vi "Control_3.vi"(0 "latd-lon-heig-VNWU":T5, 1 "CIVITA as DMARS [rad]":cluster{"phi":dbl, "theta":dbl, "psi":dbl}, 2 "Guiamento":bool, 3 "PID_array":dbl[][](array[numeric]), 5 "Wi1-Wbi1-qi1-Euli1":T6, 7 "Civita?":bool, 9 "output Rocket Dynamics":T1, 11 "File":dbl[][](array[numeric]), 12 "dt-sim_run-t-i":T4, 13 "Position (i+1)":T2, 14 "Rotation":T3, 15 "sim_running":bool) -> (4 "TVA_cmd(i+1,:) [deg]":dbl[](array[numeric]), 10 "AoA-Speed-Rocket":cluster{dbl[], dbl[], dbl[]})   [LabVIEW 2017]
uses:
  <vilib>/Analysis/coordinate.llb/Euler Rotation Order.ctl
  <vilib>/Analysis/_algsub.llb/Vector Norm Type.ctl
  <vilib>/Analysis/baseanly.llb/Real A x B.vi
  <vilib>/Analysis/_algsub.llb/Real Vector Norm.vi
  <vilib>/Analysis/Matrix/Numeric/Conversions/Array To Matrix - RA2.vi
  <vilib>/Analysis/Matrix/Numeric/Conversions/Matrix To Array - RM.vi
  <vilib>/Analysis/NI_AALPro.lvlib
  <vilib>/Analysis/Matrix/NI_Matrix.lvlib
  <vilib>/Analysis/NI_AALBase.lvlib
panel:
  out "Pitch Yaw ref [deg]":dbl[](array[numeric])
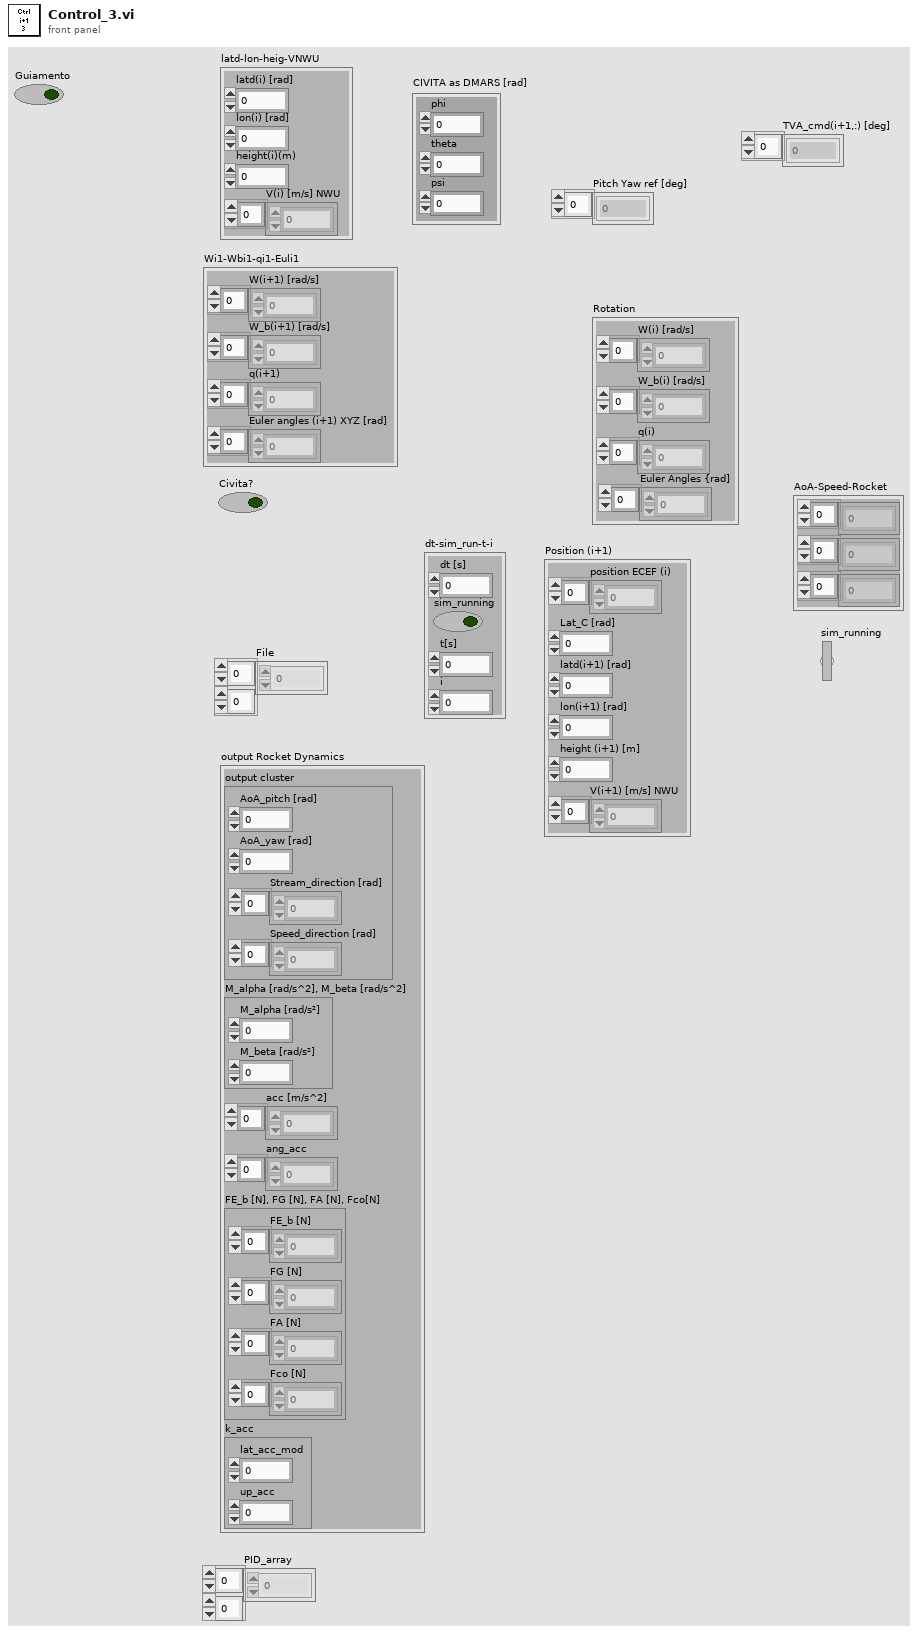
[diagram p1: front panel]
types:
  T1 = cluster{"output cluster":cluster{"AoA_pitch [rad]":dbl, "AoA_yaw [rad]":dbl, "Stream_direction [rad]":dbl[], "Speed_direction [rad]":dbl[]}, "M_alpha [rad/s^2], M_beta [rad/s^2]":cluster{"M_alpha [rad/s²]":dbl, "M_beta [rad/s²]":dbl}, "acc [m/s^2]":dbl[], "ang_acc":dbl[], "FE_b [N], FG [N], FA [N], Fco[N]":cluster{"FE_b [N]":dbl[], "FG [N]":dbl[], "FA [N]":dbl[], "Fco [N]":dbl[]}, "k_acc":cluster{"lat_acc_mod":dbl, "up_acc":dbl}}
  T2 = cluster{"position ECEF (i)":dbl[], "Lat_C [rad]":dbl, "latd(i+1) [rad]":dbl, "lon(i+1) [rad]":dbl, "height (i+1) [m]":dbl, "V(i+1) [m/s] NWU":dbl[]}
  T3 = cluster{"W(i) [rad/s]":dbl[], "W_b(i) [rad/s]":dbl[], "q(i)":dbl[], "Euler Angles {rad]":dbl[]}
  T4 = cluster{"dt [s]":dbl, "sim_running":bool, "t[s]":dbl, "i":i32}
  T5 = cluster{"latd(i) [rad]":dbl, "lon(i) [rad]":dbl, "height(i)(m)":dbl, "V(i) [m/s] NWU":dbl[]}
  T6 = cluster{"W(i+1) [rad/s]":dbl[], "W_b(i+1) [rad/s]":dbl[], "q(i+1)":dbl[], "Euler angles (i+1) XYZ [rad]":dbl[]}
  T7 = enum16{"IPD_deg_labview", "PID_deg_labview", "old 2019", "PID tunner", "VS 50 Control System database doc"}
  T8 = typedef "NI_AALPro.lvlib/Vector Norm Type.ctl" = u16
  T9 = typedef "NI_AALPro.lvlib/Euler Rotation Order.ctl" = u16
  T10 = typedef "NI_Matrix.lvlib/RealMatrix.ctl" = dbl[][]
  T11 = cluster{"M_alpha [rad/s²]":dbl, "M_beta [rad/s²]":dbl}
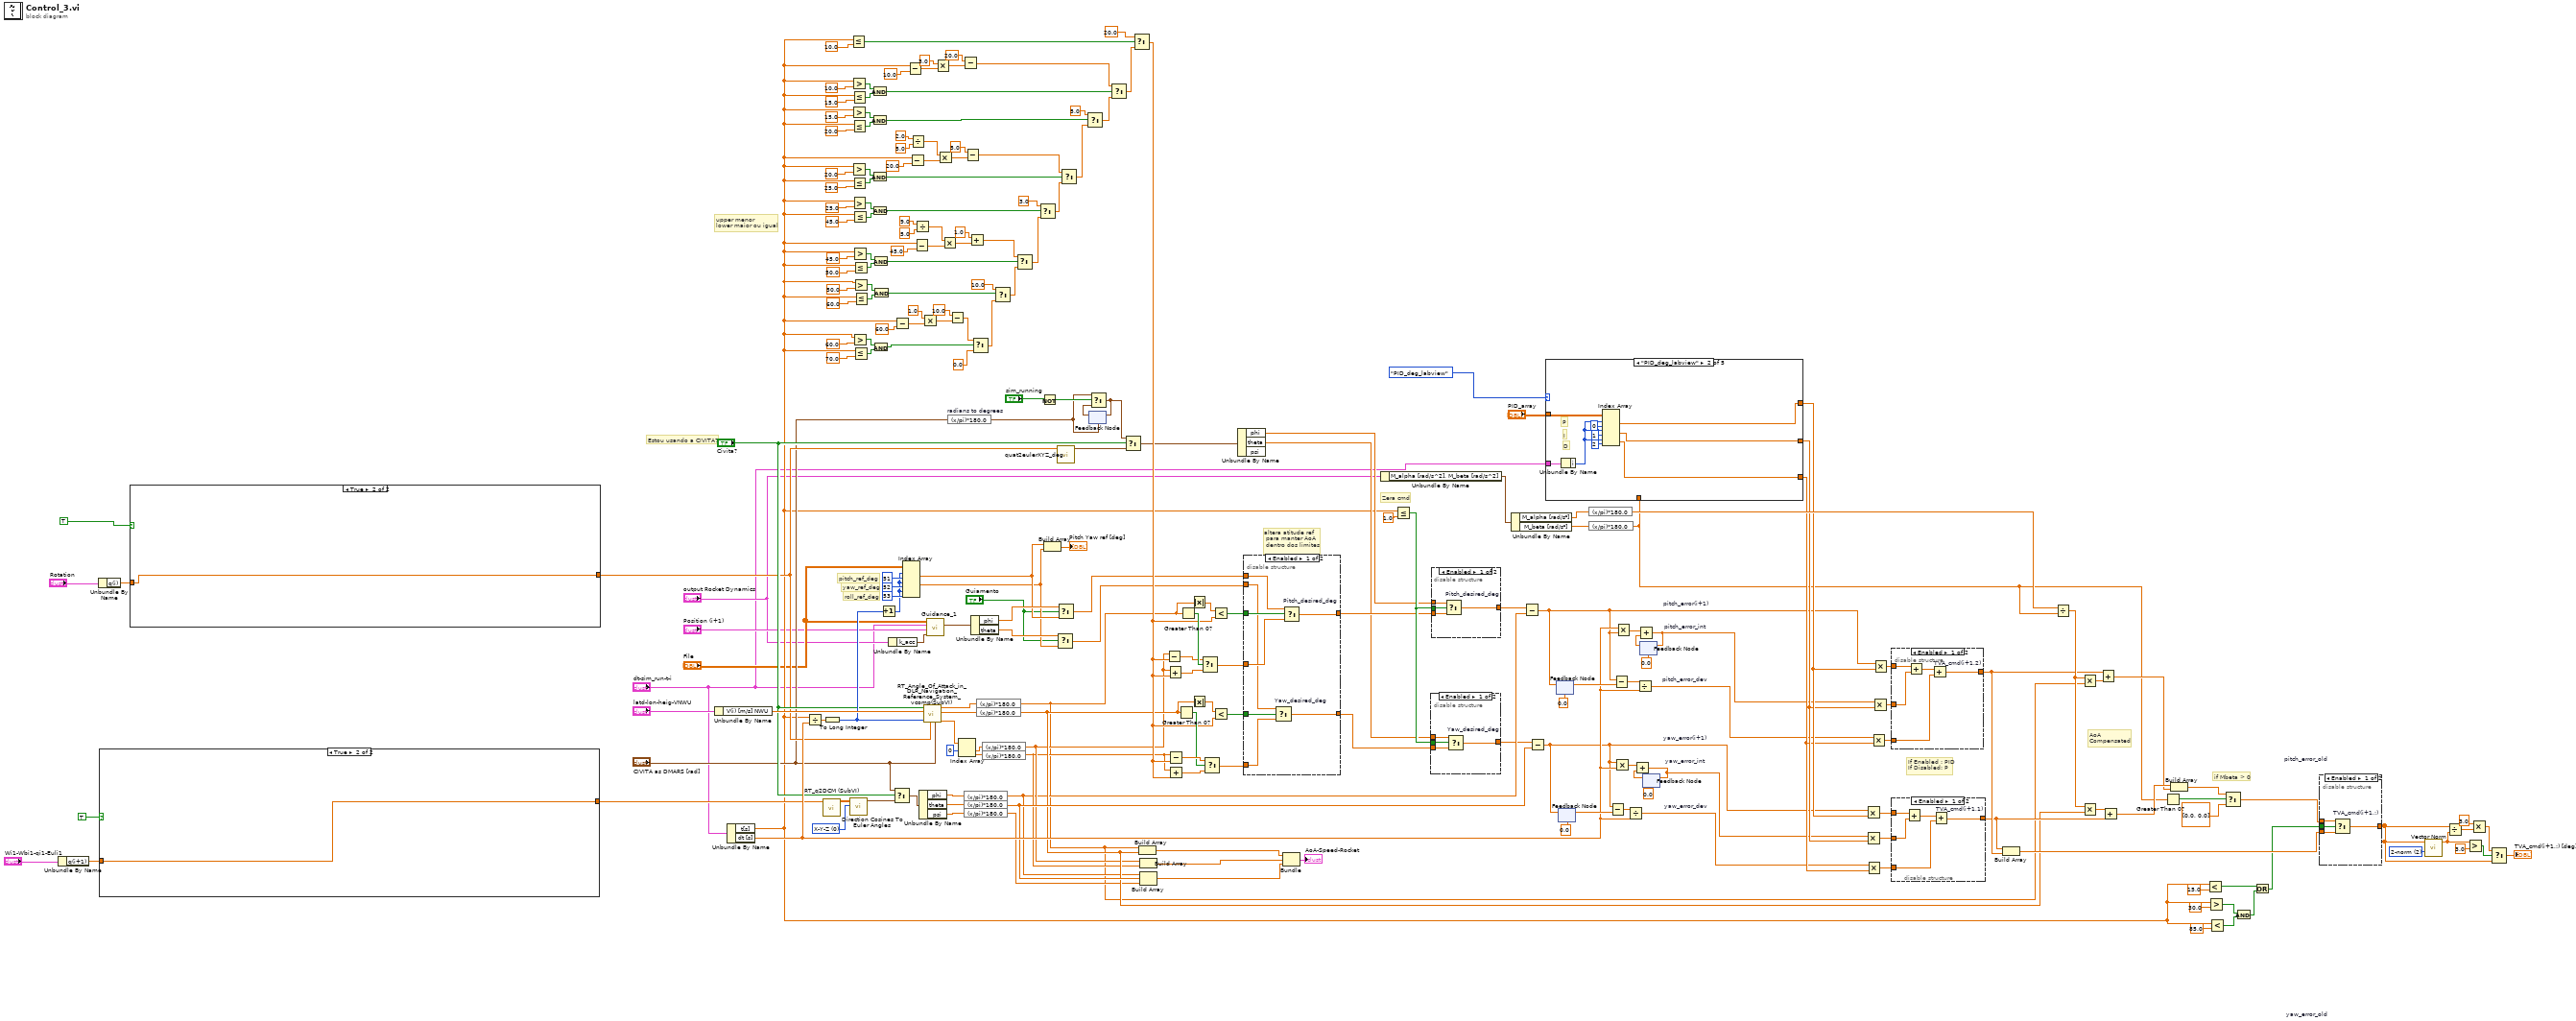
[diagram p0: block diagram]
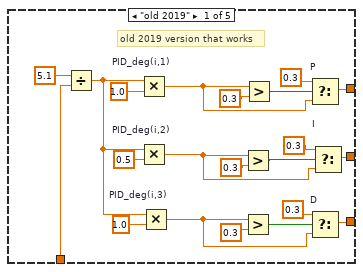
[diagram p2: hidden frame]
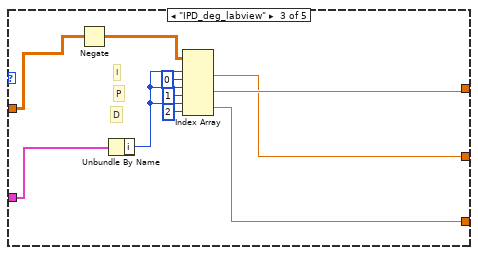
[diagram p3: hidden frame]
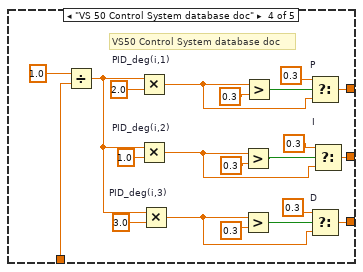
[diagram p4: hidden frame]
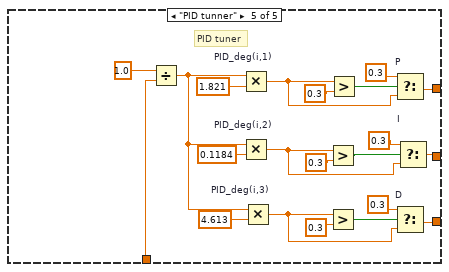
[diagram p5: hidden frame]
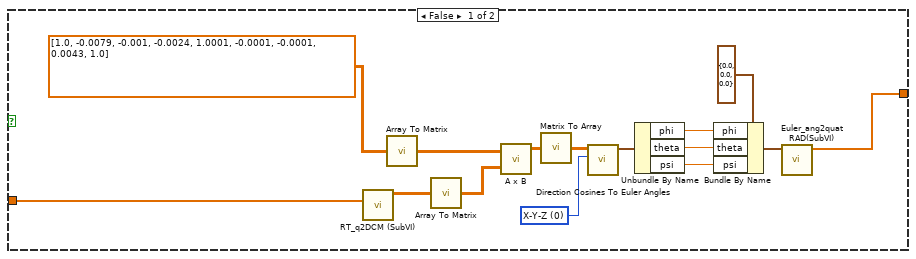
[diagram p6: hidden frame]
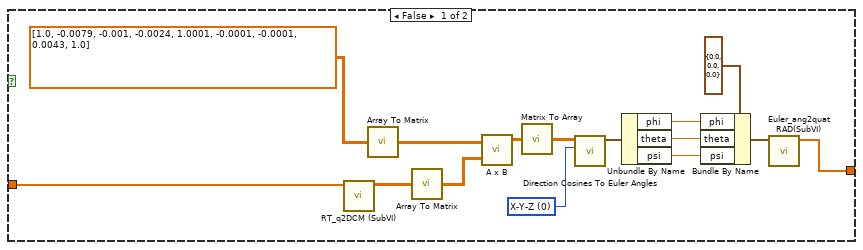
[diagram p7: hidden frame]
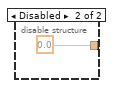
[diagram p9: hidden frame]
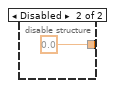
[diagram p12: hidden frame]
diagram:
  w168 = T8 2 items=["1-norm"=1, "2-norm"=2, "Inf-norm"=3, "-Inf-norm"=4, "User Defined"=5] ("norm type")
  w184 = T9 0 items=["X-Y-Z", "X-Z-Y", "Y-X-Z", "Y-Z-X", "Z-X-Y", "Z-Y-X", "X-Y-X", "X-Z-X", "Y-X-Y", "Y-Z-Y", "Z-X-Z", "Z-Y-Z"] ("rotation order")
  # "AoA\nCompensated"
  # "Estou usando a CIVITA?"
  # "If Enabled : PID\nIf Disabled: P"
  # "if Mbeta > 0"
  # "altera atitude ref\n para manter AoA\n dentro dos limites"
  # "Zera cmd"
  # "roll_ref_deg"
  # "yaw_ref_deg"
  # "pitch_ref_deg"
  # "upper menor\nlower maior ou igual"
  n1 = Unbundle By Name("Wi1-Wbi1-qi1-Euli1") -> ("q(i+1)"=w69:dbl[])
  n2 = Unbundle By Name("Rotation") -> ("q(i)"=w74:dbl[])
  n3 = case shown="True" TRUE {
    tunnel: w69 -> [w229 w242]
    tunnel: [w228 w242] -> w68
    frame False {
      w240 = T9 0 items=["X-Y-Z", "X-Z-Y", "Y-X-Z", "Y-Z-X", "Z-X-Y", "Z-Y-X", "X-Y-X", "X-Z-X", "Y-X-Y", "Y-Z-Y", "Z-X-Z", "Z-Y-Z"] ("rotation order")
      n4 = call "RT_q2DCM (SubVI).vi"("Quaternion"=w229) -> ("DCM"=w241:dbl[][])  [unwired: 10 in]
      n5 = call-poly <vilib>:"Array To Matrix.vi"("Real 2D Array"=dbl[][] [[1.0, -0.0079, -0.001], [-0.0024, 1.0001, -0.0001], [-0.0001, 0.0043, 1.0]]) -> ("Real Matrix"=w232:T10)
      n6 = call-poly <vilib>:"Array To Matrix.vi"("Real 2D Array"=w241) -> ("Real Matrix"=w231:T10)
      n7 = call-poly <vilib>:"A x B.vi"("B"=w231, "A"=w232) -> ("A x B"=w233:T10)  [unwired: 1 out]
      n8 = call-poly <vilib>:"Matrix To Array.vi"("Real Matrix"=w233) -> ("Real 2D Array"=w234:dbl[][])
      n9 = call <vilib>:"Direction Cosines To Euler Angles.vi"("rotation order"=w240, "Direction Cosines"=w234) -> ("Euler Angles"=w235:cluster{"phi":dbl, "theta":dbl, "psi":dbl})  [unwired: 8 in, 1 out]
      n10 = Unbundle By Name(w235) -> ("phi"=w238:dbl, "theta"=w239:dbl, "psi"=w227:dbl)
      n11 = Bundle By Name(cluster=cluster{"phi":dbl, "theta":dbl, "psi":dbl} {"phi"=0.0, "theta"=0.0, "psi"=0.0} ("Euler Angles 2"), "phi"=w238, "theta"=w239, "psi"=w227) -> (w236:cluster{"phi":dbl, "theta":dbl, "psi":dbl})
      n12 = call "Euler_ang2quat RAD(SubVI).vi"("Euler Angles [rad]"=w236) -> ("Quaternions"=w228:dbl[])  [unwired: 10 in]
    }
    frame True {
    }
  }
  n13 = case shown="True" TRUE {
    tunnel: w74 -> [w245 w258]
    tunnel: [w244 w258] -> w72
    frame False {
      w256 = T9 0 items=["X-Y-Z", "X-Z-Y", "Y-X-Z", "Y-Z-X", "Z-X-Y", "Z-Y-X", "X-Y-X", "X-Z-X", "Y-X-Y", "Y-Z-Y", "Z-X-Z", "Z-Y-Z"] ("rotation order")
      n14 = call "RT_q2DCM (SubVI).vi"("Quaternion"=w245) -> ("DCM"=w257:dbl[][])  [unwired: 10 in]
      n15 = call-poly <vilib>:"Array To Matrix.vi"("Real 2D Array"=dbl[][] [[1.0, -0.0079, -0.001], [-0.0024, 1.0001, -0.0001], [-0.0001, 0.0043, 1.0]]) -> ("Real Matrix"=w248:T10)
      n16 = call-poly <vilib>:"Array To Matrix.vi"("Real 2D Array"=w257) -> ("Real Matrix"=w247:T10)
      n17 = call-poly <vilib>:"A x B.vi"("B"=w247, "A"=w248) -> ("A x B"=w249:T10)  [unwired: 1 out]
      n18 = call-poly <vilib>:"Matrix To Array.vi"("Real Matrix"=w249) -> ("Real 2D Array"=w250:dbl[][])
      n19 = call <vilib>:"Direction Cosines To Euler Angles.vi"("rotation order"=w256, "Direction Cosines"=w250) -> ("Euler Angles"=w251:cluster{"phi":dbl, "theta":dbl, "psi":dbl})  [unwired: 8 in, 1 out]
      n20 = Unbundle By Name(w251) -> ("phi"=w254:dbl, "theta"=w255:dbl, "psi"=w243:dbl)
      n21 = Bundle By Name(cluster=cluster{"phi":dbl, "theta":dbl, "psi":dbl} {"phi"=0.0, "theta"=0.0, "psi"=0.0} ("Euler Angles 2"), "phi"=w254, "theta"=w255, "psi"=w243) -> (w252:cluster{"phi":dbl, "theta":dbl, "psi":dbl})
      n22 = call "Euler_ang2quat RAD(SubVI).vi"("Euler Angles [rad]"=w252) -> ("Quaternions"=w244:dbl[])  [unwired: 10 in]
    }
    frame True {
    }
  }
  n23 = Unbundle By Name("latd-lon-heig-VNWU") -> ("V(i) [m/s] NWU"=w135:dbl[])
  n24 = Unbundle By Name("dt-sim_run-t-i") -> ("t[s]"=w19:dbl, "dt [s]"=w115:dbl)
  n25 = Divide(x=w19, y=w115) -> (x/y=w191:dbl)
  n26 = call "RT_q2DCM (SubVI).vi"("Quaternion"=w68) -> ("DCM"=w185:dbl[][])  [unwired: 10 in]
  n27 = To Long Integer(number=w191) -> (32bit integer=w129:i32)
  n28 = Less Or Equal?(x=w19, y=10.0) -> (x <= y?=w225:bool)
  n29 = call <vilib>:"Direction Cosines To Euler Angles.vi"("rotation order"=w184, "Direction Cosines"=w185) -> ("Euler Angles"=w67:cluster{"phi":dbl, "theta":dbl, "psi":dbl})  [unwired: 8 in, 1 out]
  n30 = Greater?(x=w19, y=10.0) -> (0:w217:bool)
  n31 = Greater?(x=w19, y=15.0) -> (0:w213:bool)
  n32 = Greater?(x=w19, y=20.0) -> (0:w208:bool)
  n33 = Less Or Equal?(x=w19, y=15.0) -> (x <= y?=w216:bool)
  n34 = Less Or Equal?(x=w19, y=20.0) -> (x <= y?=w214:bool)
  n35 = Less Or Equal?(x=w19, y=25.0) -> (x <= y?=w207:bool)
  n36 = Greater?(x=w19, y=25.0) -> (0:w205:bool)
  n37 = Less Or Equal?(x=w19, y=45.0) -> (x <= y?=w206:bool)
  n38 = Greater?(x=w19, y=45.0) -> (0:w200:bool)
  n39 = Greater?(x=w19, y=60.0) -> (0:w55:bool)
  n40 = Less Or Equal?(x=w19, y=50.0) -> (x <= y?=w199:bool)
  n41 = Greater?(x=w19, y=50.0) -> (0:w60:bool)
  n42 = Less Or Equal?(x=w19, y=70.0) -> (x <= y?=w54:bool)
  n43 = Less Or Equal?(x=w19, y=60.0) -> (x <= y?=w61:bool)
  n44 = And(x=w217, y=w216) -> (x .and. y?=w215:bool)
  n45 = And(x=w213, y=w214) -> (x .and. y?=w198:bool)
  n46 = And(x=w208, y=w207) -> (x .and. y?=w197:bool)
  n47 = And(x=w205, y=w206) -> (x .and. y?=w195:bool)
  n48 = And(x=w200, y=w199) -> (x .and. y?=w193:bool)
  n49 = And(x=w55, y=w54) -> (x .and. y?=w48:bool)
  n50 = And(x=w60, y=w61) -> (x .and. y?=w49:bool)
  n51 = Increment(x=w129) -> (x+1=w181:i32)
  n52 = Unbundle By Name("output Rocket Dynamics") -> ("k_acc"=w8:cluster{"lat_acc_mod":dbl, "up_acc":dbl})
  n53 = Select(t="CIVITA as DMARS [rad]", s="Civita?", f=w67) -> (s? t:f=w92:cluster{"phi":dbl, "theta":dbl, "psi":dbl})
  n54 = Subtract(x=w19, y=60.0) -> (x-y=w24:dbl)
  n55 = Index Array(array="File", index (row) #1=w181, index (col) #1=51 ("disabled index (col)"), index (row) #2=w181, index (col) #2=52 ("disabled index (col)"), index (row) #3=w181, index (col) #3=53 ("disabled index (col)")) -> (element #1=w13:dbl, element #2=w11:dbl)  [unwired: 1 out]
  n56 = Subtract(x=w19, y=10.0) -> (x-y=w44:dbl)
  n57 = Subtract(x=w19, y=20.0) -> (x-y=w40:dbl)
  n58 = Divide(x=2.0 ("corr_angle_deg"), y=5.0 ("corr_angle_deg")) -> (x/y=w35:dbl)
  n59 = Subtract(x=w19, y=45.0) -> (x-y=w28:dbl)
  n60 = Divide(x=9.0 ("corr_angle_deg"), y=5.0 ("corr_angle_deg")) -> (x/y=w33:dbl)
  n61 = Unbundle By Name(w92) -> ("phi"=w183:dbl, "theta"=w182:dbl, "psi"=w96:dbl)
  n62 = Multiply(x=1.0 ("corr_angle_deg"), y=w24) -> (x*y=w25:dbl)
  n63 = call "RT_Angle_Of_Attack_in_DLR_Navigation_Reference_System_vcomp(SubVI).vi"("Euler Angles [rad]"="CIVITA as DMARS [rad]", "q"=w72, "i"=w129, "V (m/s)"=w135, "Civita?"="Civita?") -> ("Speed_direction [rad]"=w186:dbl[], "AoA_yaw (rad)"=w100:dbl, "AoA_pitch (rad)"=w101:dbl)  [unwired: 4 in]
  n64 = call "Guidance_1.vi"("k_acc"=w8, "Position (i+1)"="Position (i+1)", "Time"="dt-sim_run-t-i", "Data"="File") -> ("new_ref[deg]"=w16:cluster{"phi":dbl, "theta":dbl, "psi":dbl})  [unwired: 7 in]
  n65 = Multiply(x=3.0 ("corr_angle_deg"), y=w44) -> (x*y=w43:dbl)
  n66 = Multiply(x=w35, y=w40) -> (x*y=w41:dbl)
  n67 = Multiply(x=w33, y=w28) -> (x*y=w27:dbl)
  n68 = expression code="(x/pi)*180.0" "radians to degrees"("CIVITA as DMARS [rad]") -> (w78:cluster{"phi":dbl, "theta":dbl, "psi":dbl})
  n69 = Subtract(x=10.0 ("corr_angle_deg"), y=w25) -> (x-y=w21:dbl)
  n70 = Index Array(array=w186, index #1=0 ("index")) -> (element #1=w103:dbl, element #2=w102:dbl)  [unwired: 1 in]
  n71 = Subtract(x=20.0 ("corr_angle_deg"), y=w43) -> (x-y=w42:dbl)
  n72 = Subtract(x=5.0 ("corr_angle_deg"), y=w41) -> (x-y=w34:dbl)
  n73 = expression code="(x/pi)*180.0" ("radians to degrees")(w183) -> (w87:dbl)
  n74 = expression code="(x/pi)*180.0" ("radians to degrees")(w182) -> (w104:dbl)
  n75 = expression code="(x/pi)*180.0" ("radians to degrees")(w96) -> (w95:dbl)
  n76 = Add(x=1.0 ("corr_angle_deg"), y=w27) -> (x+y=w26:dbl)
  n77 = Unbundle By Name(w16) -> ("phi"=w15:dbl, "theta"=w14:dbl)
  n78 = Select(t=w21, s=w48, f=0.0 ("corr_angle_deg")) -> (s? t:f=w52:dbl)
  n79 = expression code="(x/pi)*180.0" ("radians to degrees")(w101) -> (w5:dbl)
  n80 = expression code="(x/pi)*180.0" ("radians to degrees")(w100) -> (w99:dbl)
  n81 = expression code="(x/pi)*180.0" ("radians to degrees")(w103) -> (w98:dbl)
  n82 = expression code="(x/pi)*180.0" ("radians to degrees")(w102) -> (w97:dbl)
  n83 = Select(t=10.0 ("corr_angle_deg"), s=w49, f=w52) -> (s? t:f=w50:dbl)
  n84 = Select(t=w26, s=w193, f=w50) -> (s? t:f=w192:dbl)
  n85 = Select(t=3.0 ("corr_angle_deg"), s=w195, f=w192) -> (s? t:f=w194:dbl)
  n86 = Not(x="sim_running") -> (.not. x?=w82:bool)
  n87 = Build Array(w13, w11) -> (→"Pitch Yaw ref [deg]":dbl[])
  n88 = Select(t=w14, s="Guiamento", f=w11) -> (s? t:f=w10:dbl)
  n89 = call "quat2eulerXYZ_deg.vi"("Quaternions"=w72) -> ("Euler Angles [deg]"=w91:cluster{"phi":dbl, "theta":dbl, "psi":dbl})  [unwired: 10 in]
  n90 = Select(t=w15, s="Guiamento", f=w13) -> (s? t:f=w12:dbl)
  n91 = Select(t=w34, s=w197, f=w194) -> (s? t:f=w220:dbl)
  n92 = Select(t=5.0 ("corr_angle_deg"), s=w198, f=w220) -> (s? t:f=w221:dbl)
  n93 = feedback #1(w78) -> (w88:cluster{"phi":dbl, "theta":dbl, "psi":dbl})
  n94 = Select(t=w78, s=w82, f=w88) -> (s? t:f=w93:cluster{"phi":dbl, "theta":dbl, "psi":dbl})
  n95 = feedback-in #1(w93) -> ()
  n96 = Select(t=w42, s=w215, f=w221) -> (s? t:f=w223:dbl)
  n97 = Select(t=w93, s="Civita?", f=w91) -> (s? t:f=w90:cluster{"phi":dbl, "theta":dbl, "psi":dbl})
  n98 = Select(t=20.0 ("corr_angle_deg"), s=w225, f=w223) -> (s? t:f=w128:dbl)
  n99 = Build Array(w5, w99) -> (w77:dbl[])
  n100 = Build Array(w98, w97) -> (w76:dbl[])
  n101 = Build Array(w87, w104, w95) -> (w75:dbl[])
  n102 = Subtract(x=w98, y=w128) -> (x-y=w156:dbl)
  n103 = Add(x=w98, y=w128) -> (x+y=w155:dbl)
  n104 = Subtract(x=w97, y=w128) -> (x-y=w153:dbl)
  n105 = Add(x=w97, y=w128) -> (x+y=w154:dbl)
  n106 = Greater Than 0?(x=w99) -> (x > 0?=w152:bool)
  n107 = Greater Than 0?(x=w5) -> (x > 0?=w157:bool)
  n108 = Absolute Value(x=w5) -> (abs(x)=w160:dbl)
  n109 = Absolute Value(x=w99) -> (abs(x)=w149:dbl)
  n110 = Select(t=w156, s=w157, f=w155) -> (s? t:f=w158:dbl)
  n111 = Select(t=w153, s=w152, f=w154) -> (s? t:f=w151:dbl)
  n112 = Less?(x=w160, y=w128) -> (x < y?=w159:bool)
  n113 = Less?(x=w149, y=w128) -> (x < y?=w150:bool)
  n114 = Unbundle By Name(w90) -> ("phi"=w80:dbl, "theta"=w79:dbl)  [unwired: 1 out]
  n115 = disable-structure shown="Enabled" {
    disable-tunnel: w10 -> [w260 w267]
    disable-tunnel: w12 -> [w262 w268]
    disable-tunnel: w159 -> [w266 _]
    disable-tunnel: w158 -> [w261 _]
    disable-tunnel: w151 -> [w259 _]
    disable-tunnel: w150 -> [w263 _]
    disable-tunnel: [w265 w268] -> w146
    disable-tunnel: [w264 w267] -> w145
    frame Enabled {
      n116 = Select "Yaw_desired_deg"(t=w260, s=w263, f=w259) -> (s? t:f=w264:dbl)
      n117 = Select "Pitch_desired_deg"(t=w262, s=w266, f=w261) -> (s? t:f=w265:dbl)
    }
    frame Disabled {
    }
  }
  n118 = Bundle(w77, w76, w75) -> (→"AoA-Speed-Rocket":cluster{dbl[], dbl[], dbl[]})  [unwired: 1 in]
  n119 = Unbundle By Name("output Rocket Dynamics") -> ("M_alpha [rad/s^2], M_beta [rad/s^2]"=w6:T11)
  n120 = Less Or Equal?(x=w19, y=1.0) -> (x <= y?=w147:bool)
  n121 = disable-structure shown="Enabled" {
    disable-tunnel: [w272 0.0 ("t")] -> w85
    disable-tunnel: w147 -> [w269 _]
    disable-tunnel: w145 -> [w271 _]
    disable-tunnel: w79 -> [w270 _]
    frame Enabled {
      n122 = Select "Yaw_desired_deg"(t=w270, s=w269, f=w271) -> (s? t:f=w272:dbl)
    }
    frame Disabled {
    }
  }
  n123 = disable-structure shown="Enabled" {
    disable-tunnel: [w277 0.0 ("t")] -> w86
    disable-tunnel: w147 -> [w276 _]
    disable-tunnel: w146 -> [w275 _]
    disable-tunnel: w80 -> [w274 _]
    frame Enabled {
      n124 = Select "Pitch_desired_deg"(t=w274, s=w276, f=w275) -> (s? t:f=w277:dbl)
    }
    frame Disabled {
    }
  }
  n125 = Unbundle By Name(w6) -> ("M_alpha [rad/s²]"=w133:dbl, "M_beta [rad/s²]"=w131:dbl)
  n126 = Subtract "pitch_error(i+1)"(x=w86, y=w87) -> (x-y=w84:dbl)
  n127 = Subtract "yaw_error(i+1)"(x=w85, y=w104) -> (x-y=w83:dbl)
  n128 = feedback #2 "pitch_error_old"(0.0) -> (w144:dbl)
  n129 = feedback-in #2(w84) -> ()
  n130 = feedback #3 "yaw_error_old"(0.0) -> (w142:dbl)
  n131 = feedback-in #3(w83) -> ()
  n132 = expression code="(x/pi)*180.0" ("radians to degrees")(w133) -> (w132:dbl)
  n133 = expression code="(x/pi)*180.0" ("radians to degrees")(w131) -> (w64:dbl)
  n134 = case shown="\"PID_deg_labview\"" T7."PID_deg_labview" {
    tunnel: [w281 w303 w313 w322 w340] -> w127
    tunnel: [w280 w302 w312 w321 w341] -> w124
    tunnel: [w279 w301 w311 w320 w342] -> w123
    tunnel: w64 -> [w282 _ _ w319 w343]
    tunnel: "dt-sim_run-t-i" -> [_ w308 w314 _ _]
    tunnel: "PID_array" -> [_ w300 w310 _ _]
    frame "old 2019" {
      # "old 2019 version that works"
      n135 = Divide(x=5.1, y=w282) -> (x/y=w295:dbl)
      n136 = Multiply "PID_deg(i,1)"(x=w295, y=1.0) -> (x*y=w291:dbl)
      n137 = Multiply "PID_deg(i,2)"(x=w295, y=0.5) -> (x*y=w286:dbl)
      n138 = Multiply "PID_deg(i,3)"(x=w295, y=1.0) -> (x*y=w285:dbl)
      n139 = Greater?(x=w286, y=0.3) -> (0:w287:bool)
      n140 = Greater?(x=w285, y=0.3) -> (0:w288:bool)
      n141 = Greater?(x=w291, y=0.3) -> (0:w293:bool)
      n142 = Select "P"(t=0.3, s=w293, f=w291) -> (s? t:f=w281:dbl)
      n143 = Select "D"(t=0.3, s=w288, f=w285) -> (s? t:f=w279:dbl)
      n144 = Select "I"(t=0.3, s=w287, f=w286) -> (s? t:f=w280:dbl)
    }
    frame "PID_deg_labview" {
      # "D"
      # "I"
      # "P"
      n145 = Unbundle By Name(w308) -> ("i"=w307:i32)
      n146 = Index Array(array=w300, index (row) #1=w307, index (col) #1=0 ("disabled index (col)"), index (row) #2=w307, index (col) #2=1 ("disabled index (col)"), index (row) #3=w307, index (col) #3=2 ("disabled index (col)")) -> (element #1=w303:dbl, element #2=w302:dbl, element #3=w301:dbl)
    }
    frame "IPD_deg_labview" {
      # "D"
      # "I"
      # "P"
      n147 = Negate(x=w310) -> (-x=w309:dbl[][])
      n148 = Unbundle By Name(w314) -> ("i"=w318:i32)
      n149 = Index Array(array=w309, index (row) #1=w318, index (col) #1=0 ("disabled index (col)"), index (row) #2=w318, index (col) #2=1 ("disabled index (col)"), index (row) #3=w318, index (col) #3=2 ("disabled index (col)")) -> (element #1=w312:dbl, element #2=w313:dbl, element #3=w311:dbl)
    }
    frame "VS 50 Control System database doc" {
      # "VS50 Control System database doc"
      n150 = Divide(x=1.0, y=w319) -> (x/y=w335:dbl)
      n151 = Multiply "PID_deg(i,1)"(x=w335, y=2.0) -> (x*y=w331:dbl)
      n152 = Multiply "PID_deg(i,2)"(x=w335, y=1.0) -> (x*y=w326:dbl)
      n153 = Multiply "PID_deg(i,3)"(x=w335, y=3.0) -> (x*y=w325:dbl)
      n154 = Greater?(x=w326, y=0.3) -> (0:w327:bool)
      n155 = Greater?(x=w325, y=0.3) -> (0:w328:bool)
      n156 = Greater?(x=w331, y=0.3) -> (0:w333:bool)
      n157 = Select "P"(t=0.3, s=w333, f=w331) -> (s? t:f=w322:dbl)
      n158 = Select "D"(t=0.3, s=w328, f=w325) -> (s? t:f=w320:dbl)
      n159 = Select "I"(t=0.3, s=w327, f=w326) -> (s? t:f=w321:dbl)
    }
    frame "PID tunner" {
      # "PID tuner"
      n160 = Divide(x=1.0, y=w343) -> (x/y=w356:dbl)
      n161 = Multiply "PID_deg(i,1)"(x=w356, y=1.821) -> (x*y=w352:dbl)
      n162 = Multiply "PID_deg(i,2)"(x=w356, y=0.1184) -> (x*y=w347:dbl)
      n163 = Multiply "PID_deg(i,3)"(x=w356, y=4.613) -> (x*y=w346:dbl)
      n164 = Greater?(x=w347, y=0.3) -> (0:w348:bool)
      n165 = Greater?(x=w346, y=0.3) -> (0:w349:bool)
      n166 = Greater?(x=w352, y=0.3) -> (0:w354:bool)
      n167 = Select "P"(t=0.3, s=w354, f=w352) -> (s? t:f=w340:dbl)
      n168 = Select "D"(t=0.3, s=w349, f=w346) -> (s? t:f=w342:dbl)
      n169 = Select "I"(t=0.3, s=w348, f=w347) -> (s? t:f=w341:dbl)
    }
  }
  n170 = Subtract ("yaw_error_dev")(x=w83, y=w142) -> (x-y=w141:dbl)
  n171 = Subtract ("pitch_error_dev")(x=w84, y=w144) -> (x-y=w143:dbl)
  n172 = Multiply(x=w83, y=w115) -> (x*y=w114:dbl)
  n173 = Multiply(x=w115, y=w84) -> (x*y=w111:dbl)
  n174 = Divide "yaw_error_dev"(x=w141, y=w115) -> (x/y=w117:dbl)
  n175 = Divide "pitch_error_dev"(x=w143, y=w115) -> (x/y=w119:dbl)
  n176 = feedback #4(0.0) -> (w112:dbl)
  n177 = Add "pitch_error_int"(x=w111, y=w112) -> (x+y=w116:dbl)
  n178 = feedback-in #4(w116) -> ()
  n179 = feedback #5(0.0) -> (w113:dbl)
  n180 = Add "yaw_error_int"(x=w114, y=w113) -> (x+y=w118:dbl)
  n181 = feedback-in #5(w118) -> ()
  n182 = Multiply(x=w83, y=w127) -> (x*y=w125:dbl)
  n183 = Multiply(x=w118, y=w124) -> (x*y=w122:dbl)
  n184 = Multiply(x=w117, y=w123) -> (x*y=w121:dbl)
  n185 = Multiply(x=w119, y=w123) -> (x*y=w126:dbl)
  n186 = Multiply(x=w116, y=w124) -> (x*y=w176:dbl)
  n187 = Multiply(x=w84, y=w127) -> (x*y=w177:dbl)
  n188 = disable-structure shown="Enabled" {
    disable-tunnel: w177 -> [w365 w366]
    disable-tunnel: w176 -> [w361 _]
    disable-tunnel: [w363 w366] -> w139
    disable-tunnel: w126 -> [w362 _]
    frame Enabled {
      n189 = Add(x=w365, y=w361) -> (x+y=w364:dbl)
      n190 = Add "TVA_cmd(i+1,2)"(x=w364, y=w362) -> (x+y=w363:dbl)
    }
    frame Disabled {
    }
  }
  n191 = disable-structure shown="Enabled" {
    disable-tunnel: w125 -> [w371 w372]
    disable-tunnel: w122 -> [w367 _]
    disable-tunnel: [w369 w372] -> w120
    disable-tunnel: w121 -> [w368 _]
    frame Enabled {
      n192 = Add(x=w371, y=w367) -> (x+y=w370:dbl)
      n193 = Add "TVA_cmd(i+1,1)"(x=w370, y=w368) -> (x+y=w369:dbl)
    }
    frame Disabled {
    }
  }
  n194 = Build Array(w120, w139) -> (w106:dbl[])
  n195 = Divide(x=w132, y=w64) -> (x/y=w170:dbl)
  n196 = Multiply(x=w170, y=w5) -> (x*y=w63:dbl)
  n197 = Multiply(x=w170, y=w99) -> (x*y=w62:dbl)
  n198 = Add(x=w139, y=w63) -> (x+y=w137:dbl)
  n199 = Add(x=w62, y=w120) -> (x+y=w138:dbl)
  n200 = Greater Than 0?(x=w64) -> (x > 0?=w172:bool)
  n201 = Build Array(w138, w137) -> (w169:dbl[])
  n202 = Less?(x=w19, y=15.0) -> (x < y?=w108:bool)
  n203 = Greater?(x=w19, y=30.0) -> (0:w110:bool)
  n204 = Less?(x=w19, y=85.0) -> (x < y?=w109:bool)
  n205 = Select(t=w169, s=w172, f=dbl[] [0.0, 0.0] ("appended array")) -> (s? t:f=w130:dbl[])
  n206 = And(x=w110, y=w109) -> (x .and. y?=w107:bool)
  n207 = Or(x=w108, y=w107) -> (x .or. y?=w4:bool)
  n208 = disable-structure shown="Enabled" {
    disable-tunnel: w4 -> [w376 _]
    disable-tunnel: w130 -> [w375 _]
    disable-tunnel: w106 -> [w374 w377]
    disable-tunnel: [w373 w377] -> w140
    frame Enabled {
      n209 = Select "TVA_cmd(i+1,:)"(t=w375, s=w376, f=w374) -> (s? t:f=w373:dbl[])
    }
    frame Disabled {
    }
  }
  n210 = call-poly <vilib>:"Vector Norm.vi"("norm type"=w168, "Input Vector"=w140) -> ("norm"=w165:dbl)  [unwired: 8 in, 1 out]
  n211 = Divide(x=w140, y=w165) -> (x/y=w163:dbl[])
  n212 = Greater?(x=w165, y=3.0) -> (0:w166:bool)
  n213 = Multiply(x=3.0, y=w163) -> (x*y=w162:dbl[])
  n214 = Select(t=w162, s=w166, f=w140) -> (s? t:f=→"TVA_cmd(i+1,:) [deg]":dbl[])
